vi "Get This Application.vi"(11 "TEMPLATE Queue in":refnum<class "TEMPLATE Queue.lvclass">) -> (2 "This Application":refnum<vi>)   [LabVIEW 2021, in "_Template.lvlib" / "Templates.lvlib" / "TEMPLATE Queue.lvlib" / "TEMPLATE Queue.lvclass"]
uses:
  TEMPLATE Queue.lvclass
  TEMPLATE Queue.lvclass/TEMPLATE Queue.ctl
  jettl/jettl/Queue/Queue.lvclass
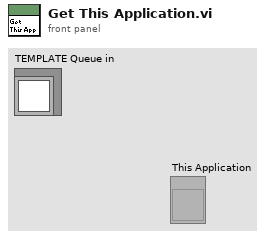
[diagram p1: front panel]
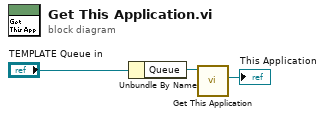
[diagram p0: block diagram]
diagram:
  n1 = Unbundle By Name("TEMPLATE Queue in") -> ("Queue"=w2:refnum<class "Queue.lvclass">)
  n2 = call-dynamic "Get This Application.vi"("jettl in"=w2) -> ("This Application"=→"This Application":refnum<vi>)  [unwired: 10 in]
